vi "Ensure Load Measurements Exists.vi"(7 "Bus by ID":T1[](array[typedef]), 10 "Load Power Measurements":dbl[](array[numeric]), 11 "Generic Optimization in":refnum<class "Generic Optimization.lvclass">) -> (2 "Load Power Measurements":dbl[](array[numeric]))   [LabVIEW 2018, in "Generic Optimization Actor.lvlib" / "Generic Optimization.lvclass"]
uses:
  Generic Optimization.lvclass
  C:/Users/Administrator/Desktop/LabVIEW EMS/EMS Generic Actor/EMS Generic/EMS Generic.lvclass
  Optimization Controls/Bus by ID.ctl
  <vilib>/ORNL/CSEISMIC DDS/CSEISMIC DDS Base/Data Types/Controls/DeviceID.ctl
  EMS Generic Actor/EMS Generic/EMS Generic.lvclass/EMS Generic.ctl
  <vilib>/ORNL/CSEISMIC DDS/CSEISMIC DDS Base/Data Types/SmartRelay_Measurement.ctl
  EMS Generic Actor/EMS Generic/EMS Generic.lvclass
  <vilib>/ORNL/CSEISMIC DDS/CSEISMIC DDS Base/CSEISMIC DDS.lvclass
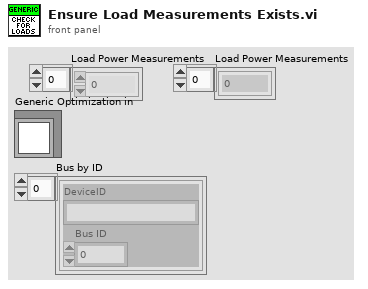
[diagram p1: front panel]
types:
  T1 = typedef "Generic Optimization Actor.lvlib/Generic Optimization.lvclass/Bus by ID.ctl" = cluster{"DeviceID":T2, "Bus ID":dbl}
  T2 = typedef "CSEISMIC DDS.lvlib/CSEISMIC DDS.lvclass/DeviceID.ctl" = string
  T3 = typedef "CSEISMIC DDS.lvlib/CSEISMIC DDS.lvclass/SmartRelay_Measurement.ctl" = cluster{"DeviceID":T2, "PrimaryVoltage":dbl[], "SecondaryVoltage":dbl[], "Current":dbl[], "RealPower":dbl[], "ReactivePower":dbl[], "LineConfig":u8[], "Frequency":dbl}
  T4 = typedef "EMS Generic Actor.lvlib/EMS Generic.lvclass/Data Type DVRs.ctl" = cluster{"IED_Status":refnum<data-value>, "IED_Status_0":refnum<data-value>, "DER_Measurement":refnum<data-value>, "DER_Info":refnum<data-value>, "DER_Status":refnum<data-value>, "ES_Measurement":refnum<data-value>, "ES_Info":refnum<data-value>, "PV_Info":refnum<data-value>, "SmartRelay_Info":refnum<data-value>, "SmartRelay_Measurement":refnum<data-value>, "Meter_Info":refnum<data-value>, "Meter_Measurement":refnum<data-value>, "HVAC_Status":refnum<data-value>, "HVAC_Measurement":refnum<data-value>, "PriceData_RealTime":refnum<data-value>, "PriceData_Demand":refnum<data-value>, "PriceData_Energy":refnum<data-value>, "ForecastData_Long":refnum<data-value>, "ForecastData_Short":refnum<data-value>, "DER_Control":refnum<data-value>, "DER_SetPointF":refnum<data-value>, "DER_SetPointP":refnum<data-value>, "DER_SetPointQ":refnum<data-value>, "DER_SetPointPF":refnum<data-value>, "DER_SetPointV":refnum<data-value>, "PV_setCurtailment":refnum<data-value>, "PV_setRampRate":refnum<data-value>, "Relay_Control":refnum<data-value>, "Load_Control":refnum<data-value>, "HVAC_Control":refnum<data-value>, "Generator_Info":refnum<data-value>, "ForecastData_Long_Backup":refnum<data-value>, "PriceData_RealTime_Backup":refnum<data-value>}
  T5 = typedef "CSEISMIC DDS.lvlib/CSEISMIC DDS.lvclass/ForecastData_Data.ctl" = cluster{"DeviceID":T2, "TargetID":T2, "t0":dbl, "dt":dbl, "Magnitude":dbl[]}
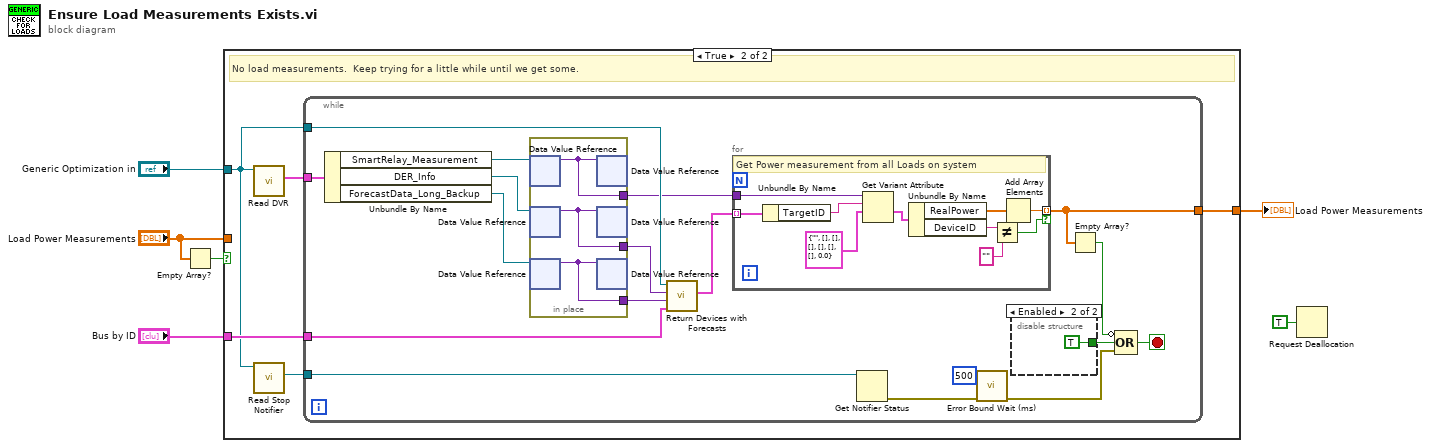
[diagram p0: block diagram]
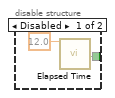
[diagram p3: hidden frame]
diagram:
  n1 = Empty Array?(array="Load Power Measurements") -> (empty?=w5:bool)
  n2 = case shown="True" w5 {
    tunnel: "Load Power Measurements" -> [w7 _]
    tunnel: "Generic Optimization in" -> [_ w9]
    tunnel: "Bus by ID" -> [_ w11]
    tunnel: [w7 w10] -> w2
    frame False {
      # "Load measurements present.  Pass the data through."
    }
    frame True {
      # "No load measurements.  Keep trying for a little while until we get some."
      n3 = call "Read DVR.vi"("EMS Generic in"=w9) -> ("DVR"=w12:T4)  [unwired: 9 in, 1 out]
      n4 = call "Read Stop Notifier.vi"("EMS Generic in"=w9) -> ("stop"=w8:refnum<notifier>)  [unwired: 9 in, 1 out]
      n5 = while {
        tunnel: w12 -> [w30]
        tunnel: w11 -> [w21]
        tunnel: [w25] -> w10
        tunnel: w9 -> [w18]
        tunnel: w8 -> [w16]
        stop <- w22 stop-if-true
        n6 = Unbundle By Name(w30) -> ("SmartRelay_Measurement"=w29:refnum<data-value>, "DER_Info"=w28:refnum<data-value>, "ForecastData_Long_Backup"=w27:refnum<data-value>)
        n7 = in-place {
          in-place-border: [w36] -> w20
          in-place-border: [w35] -> w19
          in-place-border: [w34] -> w17
          n8 = in-place-dvr #1(w29) -> (w34:variant)  [unwired: 1 out]
          n9 = in-place-dvr #2(w28) -> (w35:variant)  [unwired: 1 out]
          n10 = in-place-dvr #3(w27) -> (w36:variant)  [unwired: 1 out]
          n11 = in-place-dvr #1(w34) -> ()  [unwired: 2 out]
          n12 = in-place-dvr #2(w35) -> ()  [unwired: 2 out]
          n13 = in-place-dvr #3(w36) -> ()  [unwired: 2 out]
        }
        n14 = call "Return Devices with Forecasts.vi"("Bus by ID"=w21, "ForecastData_Long"=w20, "DER_Info"=w19, "Generic Optimization in"=w18) -> ("Forecasts with Devices"=w26:T5[])  [unwired: 4 in, 3 out]
        n15 = for {
          tunnel: w26 -> [w46] mode=indexing
          tunnel: w17 -> [w45]
          tunnel: [w42] -> w25 mode=indexing if=w38
          # "Get Power measurement from all Loads on system"
          n16 = Unbundle By Name(w46) -> ("TargetID"=w37:T2)
          n17 = Get Variant Attribute(Variant=w45, name=w37, default value (empty Variant)=T3 {"DeviceID"="", "PrimaryVoltage"=[], "SecondaryVoltage"=[], "Current"=[], "RealPower"=[], "ReactivePower"=[], "LineConfig"=[], "Frequency"=0.0} ("SmartRelay_Measurement")) -> (value=w44:T3)  [unwired: 1 in, 3 out]
          n18 = Unbundle By Name(w44) -> ("RealPower"=w41:dbl[], "DeviceID"=w39:T2)
          n19 = Not Equal?(x=w39, y=T2 "") -> (x != y?=w38:bool)
          n20 = Add Array Elements(numeric array=w41) -> (sum=w42:dbl)
        }
        n21 = Get Notifier Status(notifier=w16) -> (error out=w15:errorcluster)  [unwired: 1 in, 4 out]
        n22 = call "Error Bound Wait (ms).vi"("milliseconds to wait (100)"=u32 500 ("milliseconds to wait"), "error in"=w15) -> ("error out"=w14:errorcluster)  [unwired: 9 in]
        n23 = disable-structure shown="Enabled" {
          disable-tunnel: [w31 TRUE ("Time has Elapsed")] -> w23
          frame Disabled {
            n24 = call "Elapsed Time"("Time Target (s)"=12.0) -> ("Time has Elapsed"=w31:bool)  [unwired: 11 in, 7 out]
          }
          frame Enabled {
          }
        }
        n25 = Empty Array?(array=w25) -> (empty?=w24:bool)
        n26 = Compound Arithmetic op=OR(invert w24, w23, w14) -> (w22:bool)
      }
    }
  }
  "Load Power Measurements" <- w2
  n27 = Request Deallocation(TRUE ("flag")) -> ()
